vi "MainStatus.vi"(10 "Port":string, 11 "IP":string) -> (3 "Output All":string)   [LabVIEW 2015]
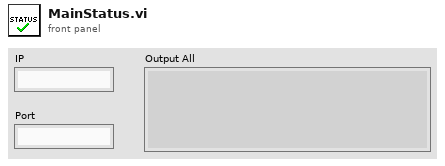
[diagram p1: front panel]
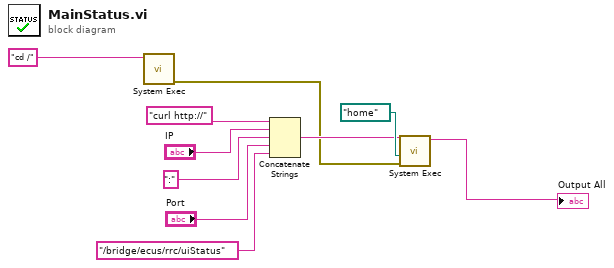
[diagram p0: block diagram]
diagram:
  n1 = call <vilib>:"System Exec.vi"("command line"="cd /") -> ("error out"=w2:errorcluster)  [unwired: 7 in, 3 out]
  n2 = Concatenate Strings("curl http://" ("string"), "IP", ":" ("string"), "Port", "/bridge/ecus/rrc/uiStatus" ("string")) -> (w8:string)
  n3 = call <vilib>:"System Exec.vi"("error in (no error)"=w2, "working directory"=path "/home", "command line"=w8) -> ("standard output"=→"Output All":string)  [unwired: 5 in, 3 out]
